vi "AlliGator Compute Decay Average Lifetime.vi"(6 "Average Lifetime Options":T1 {"Baseline %" min=0.0 max=100.0}, 8 "error in (no error)":errorcluster, 9 "t_0_IRF":dbl, 10 "<tau>_IRF":dbl, 11 "Plot":cluster{"X Array":dbl[], "Y Array":dbl[]}) -> (0 "error out":errorcluster, 3 "Average Lifetime Outputs":dbl[](array[numeric]))   [LabVIEW 2021, in "AlliGator Decay Processing.lvlib"]
doc: "Computes an estimate of the average lifetime of a decay using the formula <tau > = <tau >_F_T - <tau >_IRF_T where F_T is the decay and IRF_T is the IRF.\n\nThis calculation involves estimating the location of the rising time for both IRF and decay.\n\nWhen the option \"Use Local IRF\" is selected and a <B>Decay Location</B> is provided, the corresponding local IRF (if it exists) is used."
uses:
  AlliGator Decay Processing.lvlib
  <vilib>/Analysis/2dsp.llb/Integral Method.ctl
  Settings/AlliGator Average Lifetime Options.ctl
  Graphs/XY Graph/XY Graph Add-Ons.lvlib
  <vilib>/Analysis/NI_AALPro.lvlib
  <vilib>/Analysis/8numeric.llb/1D Numeric Integration.vi
  Settings/AlliGator Settings.lvlib
panel:
  out "[<tau_F>]":dbl[](array[numeric])
  in  "integration method":T2 items=["Trapezoidal Rule", "Simpson's Rule", "Simpson's 3/8 Rule", "Bode Rule"]
  # "<tau>, <tau)_F, t_0_F, <tau>_IRF, t_0_IRF"
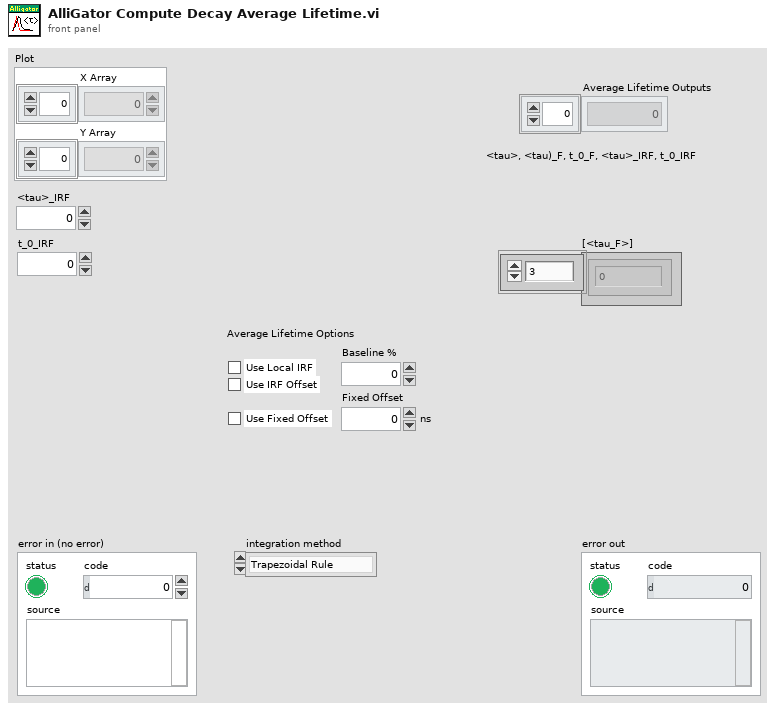
[diagram p1: front panel]
types:
  T1 = typedef "AlliGator Settings.lvlib/AlliGator Average Lifetime Options.ctl" = cluster{"Use Local IRF ":bool, "Use IRF Offset":bool, "Use Fixed Offset":bool, "Fixed Offset":dbl[unit], "Baseline %":dbl}
  T2 = typedef "NI_AALPro.lvlib/Integral Method.ctl" = i32
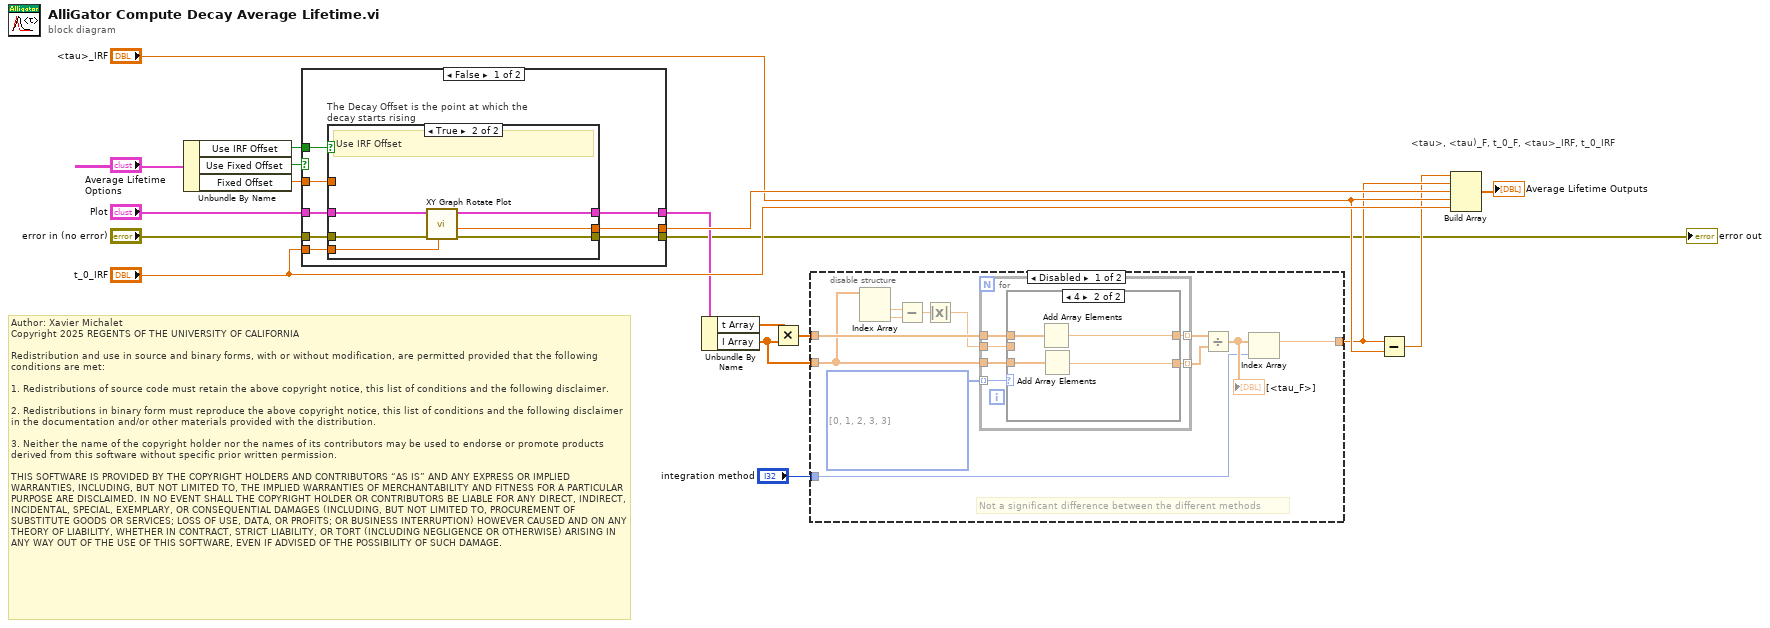
[diagram p0: block diagram]
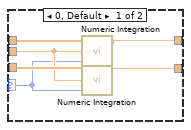
[diagram p2: hidden frame]
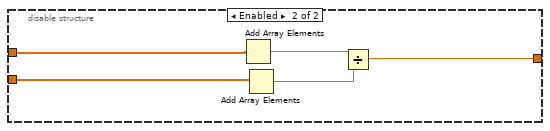
[diagram p3: hidden frame]
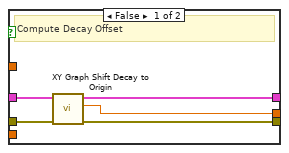
[diagram p4: hidden frame]
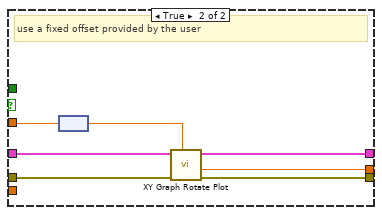
[diagram p5: hidden frame]
diagram:
  # "Author: Xavier Michalet\nCopyright 2025 REGENTS OF THE UNIVERSITY OF CALIFORNIA\n\nRedistribution and use in source and binary forms, with or without modification, are permitted provided that the following conditions are met:\n\n1. Redistributions of source code must retain the above copyright notice, this list of conditions and the following disclaimer.\n\n2. Redistributions in binary form must reproduce the above copyright notice, this list of conditions and the following disclaimer in the documentation and/or other materials provided with the distribution.\n\n3. Neither the name of the copyright holder nor the names of its contributors may be used to endorse or promote products derived from this software without specific prior written permission.\n\nTHIS SOFTWARE IS PROVIDED BY THE COPYRIGHT HOLDERS AND CONTRIBUTORS “AS IS” AND ANY EXPRESS OR IMPLIED WARRANTIES, INCLUDING, BUT NOT LIMITED TO, THE IMPLIED WARRANTIES OF MERCHANTABILITY AND FITNESS FOR A PARTICULAR PURPOSE ARE DISCLAIMED. IN NO EVENT SHALL THE COPYRIGHT HOLDER OR CONTRIBUTORS BE LIABLE FOR ANY DIRECT, INDIRECT, INCIDENTAL, SPECIAL, EXEMPLARY, OR CONSEQUENTIAL DAMAGES (INCLUDING, BUT NOT LIMITED TO, PROCUREMENT OF SUBSTITUTE GOODS OR SERVICES; LOSS OF USE, DATA, OR PROFITS; OR BUSINESS INTERRUPTION) HOWEVER CAUSED AND ON ANY THEORY OF LIABILITY, WHETHER IN CONTRACT, STRICT LIABILITY, OR TORT (INCLUDING NEGLIGENCE OR OTHERWISE) ARISING IN ANY WAY OUT OF THE USE OF THIS SOFTWARE, EVEN IF ADVISED OF THE POSSIBILITY OF SUCH DAMAGE."
  # "<tau>, <tau)_F, t_0_F, <tau>_IRF, t_0_IRF"
  n1 = Unbundle By Name("Average Lifetime Options") -> ("Use IRF Offset"=w4:bool, "Use Fixed Offset"=w7:bool, "Fixed Offset"=w8:dbl[unit])
  n2 = case shown="False" w7 {
    tunnel: w4 -> [w26 _]
    tunnel: "Plot" -> [w25 w43]
    tunnel: "error in (no error)" -> [w24 w42]
    tunnel: [w23 w41] -> w6
    tunnel: "t_0_IRF" -> [w22 _]
    tunnel: [w21 w40] -> w16
    tunnel: w8 -> [w20 w38]
    tunnel: [w19 w39] -> w9
    frame False {
      n3 = case "The Decay Offset is the point at which the decay starts rising" shown="True" w26 {
        tunnel: w22 -> [_ w36]
        tunnel: [w29 w36] -> w21
        tunnel: w25 -> [w31 w35]
        tunnel: w24 -> [w30 w33]
        tunnel: [w28 w32] -> w23
        tunnel: w20 -> [_ _]
        tunnel: [w27 w34] -> w19
        frame False {
          # "Compute Decay Offset"
          n4 = call "XY Graph Shift Decay to Origin.vi"("error in (no error)"=w30, "Decay in"=w31) -> ("error out"=w28:errorcluster, "t_0"=w29:dbl, "Rotated Decay out"=w27:cluster{"t Array":dbl[], "I Array":dbl[]})  [unwired: 6 in, 1 out]
        }
        frame True {
          # "Use IRF Offset"
          n5 = call "XY Graph Rotate Plot.vi"("t_0 (NaN: use index)"=w36, "Error In"=w33, "Decay in"=w35) -> ("Error Out"=w32:errorcluster, "Decay out"=w34:cluster{"t Array":dbl[], "I Array":dbl[]})  [unwired: 6 in, 1 out]
        }
      }
    }
    frame True {
      # "use a fixed offset provided by the user"
      n6 = node(w38) -> (w37:dbl)
      n7 = call "XY Graph Rotate Plot.vi"("t_0 (NaN: use index)"=w37, "Error In"=w42, "Decay in"=w43) -> ("Error Out"=w41:errorcluster, "t_0"=w40:dbl, "Decay out"=w39:cluster{"t Array":dbl[], "I Array":dbl[]})  [unwired: 6 in]
    }
  }
  "error out" <- w6
  n8 = Unbundle By Name(w9) -> ("t Array"=w11:dbl[], "I Array"=w1:dbl[])
  n9 = Multiply(x=w11, y=w1) -> (x*y=w2:dbl[])
  n10 = disable-structure shown="Disabled" {
    disable-tunnel: w1 -> [w44 w75]
    disable-tunnel: w2 -> [w55 w76]
    disable-tunnel: [w46 w72] -> w14
    disable-tunnel: "integration method" -> [w45 _]
    frame Disabled {
      w51 = T2[] [0, 1, 2, 3, 3] items=["Trapezoidal Rule", "Simpson's Rule", "Simpson's 3/8 Rule", "Bode Rule"] ("Array")
      # "Not a significant difference between the different methods"
      n11 = Index Array(array=w44) -> (element #1=w50:dbl, element #2=w49:dbl)  [unwired: 2 in]
      n12 = Subtract(x=w50, y=w49) -> (x-y=w48:dbl)
      n13 = Absolute Value(x=w48) -> (abs(x)=w47:dbl)
      n14 = for {
        tunnel: w44 -> [w61]
        tunnel: w55 -> [w60]
        tunnel: [w59] -> w54 mode=indexing
        tunnel: [w58] -> w53 mode=indexing
        tunnel: w51 -> [w57] mode=indexing
        tunnel: w47 -> [w56]
        n15 = case shown="4" w57 {
          selector: w57 -> [w62 _]
          tunnel: w61 -> [w65 w71]
          tunnel: w60 -> [w67 w70]
          tunnel: [w66 w69] -> w59
          tunnel: [w64 w68] -> w58
          tunnel: w56 -> [w63 _]
          frame 0, Default {
            n16 = call-poly <vilib>:"Numeric Integration.vi"("integration method"=w62, "dt"=w63, "Input Array"=w67) -> ("result"=w66:dbl)  [unwired: 1 out]
            n17 = call-poly <vilib>:"Numeric Integration.vi"("integration method"=w62, "dt"=w63, "Input Array"=w65) -> ("result"=w64:dbl)  [unwired: 1 out]
          }
          frame 4 {
            n18 = Add Array Elements(numeric array=w70) -> (sum=w69:dbl)
            n19 = Add Array Elements(numeric array=w71) -> (sum=w68:dbl)
          }
        }
      }
      n20 = Divide(x=w54, y=w53) -> (x/y=w52:dbl[])
      "[<tau_F>]" <- w52
      n21 = Index Array(array=w52, index=w45) -> (element=w46:dbl)
    }
    frame Enabled {
      n22 = Add Array Elements(numeric array=w76) -> (sum=w74:dbl)
      n23 = Add Array Elements(numeric array=w75) -> (sum=w73:dbl)
      n24 = Divide(x=w74, y=w73) -> (x/y=w72:dbl)
    }
  }
  n25 = Subtract(x=w14, y="<tau>_IRF") -> (x-y=w13:dbl)
  n26 = Build Array(w13, w14, w16, "<tau>_IRF", "t_0_IRF") -> (→"Average Lifetime Outputs":dbl[])
